vi "GEN_TimerPerS.vi"(9 "Data_In":T1 {"GUI Data Cluster"."SBR" format="%08b"}, 10 "Config_In":T3={"General"={"Config.ini"=path "", "Default Logging Path"=path ""}, "Hardware"={"Global T VAR"="", "Global B VAR"="", "VISAS"={"GEN COM"="", "SCOPE COM"="", "VNA COM"=""}, "Connected?"={"SCOPE"=FALSE, "GEN"=FALSE, "VNA"=FALSE}}, "Operation"={"Operation Mode"=enum."Idle-Off", "Status"="", "NewLog?"=FALSE, "OvenWarn"=FALSE, "Scope Settings"={"TimeBase"=0.0, "VerticalScale"=4.0, "Channel"=enum."Channel 2"}, "Gen Settings"={"Amplitude"=0.0, "Frequency"=0.0, "Offset"=0.0}}}) -> (0 "Time":bool, 1 "Data_In 2":T1 {"GUI Data Cluster"."SBR" format="%08b"}, 2 "Config_In 2":T3={"General"={"Config.ini"=path "", "Default Logging Path"=path ""}, "Hardware"={"Global T VAR"="", "Global B VAR"="", "VISAS"={"GEN COM"="", "SCOPE COM"="", "VNA COM"=""}, "Connected?"={"SCOPE"=FALSE, "GEN"=FALSE, "VNA"=FALSE}}, "Operation"={"Operation Mode"=enum."Idle-Off", "Status"="", "NewLog?"=FALSE, "OvenWarn"=FALSE, "Scope Settings"={"TimeBase"=0.0, "VerticalScale"=4.0, "Channel"=enum."Channel 2"}, "Gen Settings"={"Amplitude"=0.0, "Frequency"=0.0, "Offset"=0.0}}})   [LabVIEW 2021]
uses:
  Data_Cluster.ctl
  Measurement_Cluster.ctl
  Config_Cluster.ctl
  Mode_Enum.ctl
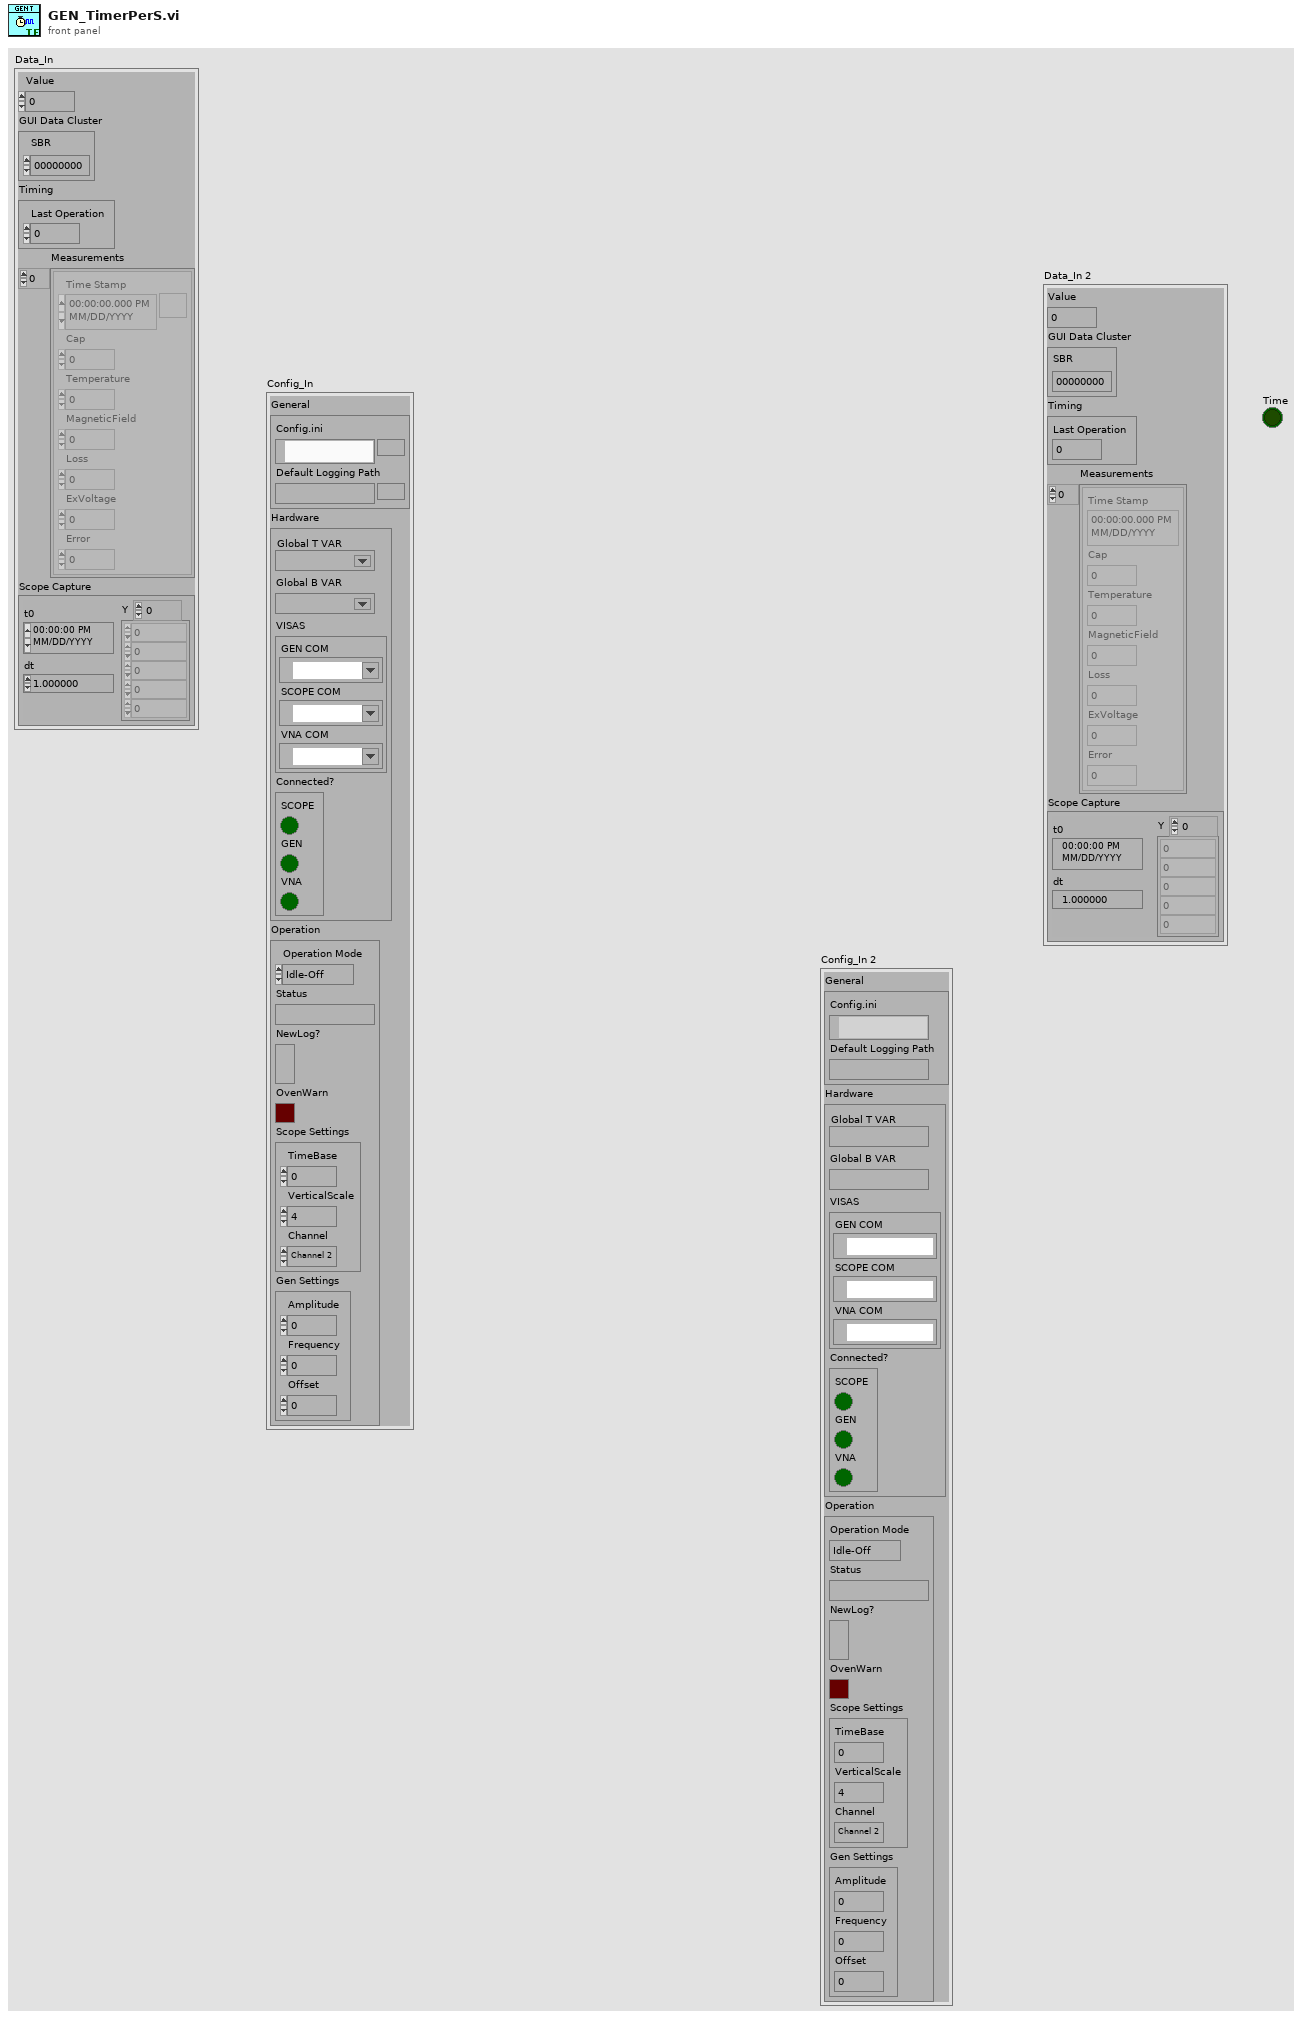
[diagram p1: front panel]
types:
  T1 = typedef "Data_Cluster.ctl" = cluster{"Value":dbl, "GUI Data Cluster":cluster{"SBR":u16}, "Timing":cluster{"Last Operation":dbl}, "Measurements":T2[], "Scope Capture":waveform(dbl)}
  T2 = typedef "Measurement_Cluster.ctl" = cluster{"Time Stamp":timestamp, "Cap":dbl, "Temperature":dbl, "MagneticField":dbl, "Loss":dbl, "ExVoltage":dbl, "Error":dbl}
  T3 = typedef "Config_Cluster.ctl" = cluster{"General":cluster{"Config.ini":path, "Default Logging Path":path}, "Hardware":cluster{"Global T VAR":refnum<k21>, "Global B VAR":refnum<k21>, "VISAS":cluster{"GEN COM":refnum<visa-resource-name>, "SCOPE COM":refnum<visa-resource-name>, "VNA COM":refnum<visa-resource-name>}, "Connected?":cluster{"SCOPE":bool, "GEN":bool, "VNA":bool}}, "Operation":cluster{"Operation Mode":T4, "Status":string, "NewLog?":bool, "OvenWarn":bool, "Scope Settings":cluster{"TimeBase":dbl, "VerticalScale":dbl, "Channel":enum16{"Channel 2", "Channel 1"}}, "Gen Settings":cluster{"Amplitude":dbl, "Frequency":dbl, "Offset":dbl}}}
  T4 = typedef "Mode_Enum.ctl" = enum16{"Logging", "Idle-Off", "Idle"}
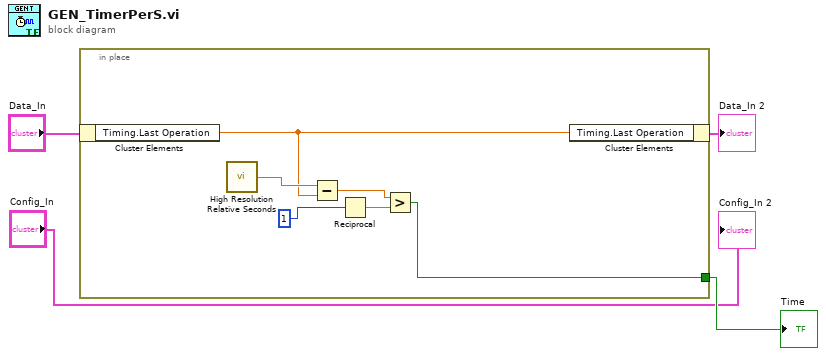
[diagram p0: block diagram]
diagram:
  n1 = in-place {
    in-place-border: [w6] -> w2
    n2 = in-place-cluster #1("Data_In") -> ("Timing.Last Operation"=w9:dbl)
    n3 = call <vilib>:"High Resolution Relative Seconds.vi"() -> ("relative seconds"=w10:dbl)
    n4 = Subtract(x=w10, y=w9) -> (x-y=w7:dbl)
    n5 = Reciprocal(x=1) -> (1/x=w8:dbl)
    n6 = Greater?(x=w7, y=w8) -> (0:w6:bool)
    n7 = in-place-cluster #1("Timing.Last Operation"=w9) -> (→"Data_In 2":T1)
  }
  "Time" <- w2
  "Config_In 2" <- "Config_In"
